vi "terminate.vi"(8 "error in (no error)":errorcluster, 11 "ExperimentControllerDL090803Triggered in":refnum<class "ExperimentControllerDL090803Triggered.lvclass">) -> (0 "error out":errorcluster, 3 "ExperimentControllerDL090803Triggered out":refnum<class "ExperimentControllerDL090803Triggered.lvclass">)   [LabVIEW 2010]
doc: "The dynamic dispatch version of this VI terminates the plug-in object by releasing all of its resources."
uses:
  ExperimentControllerDL090803Triggered.lvclass
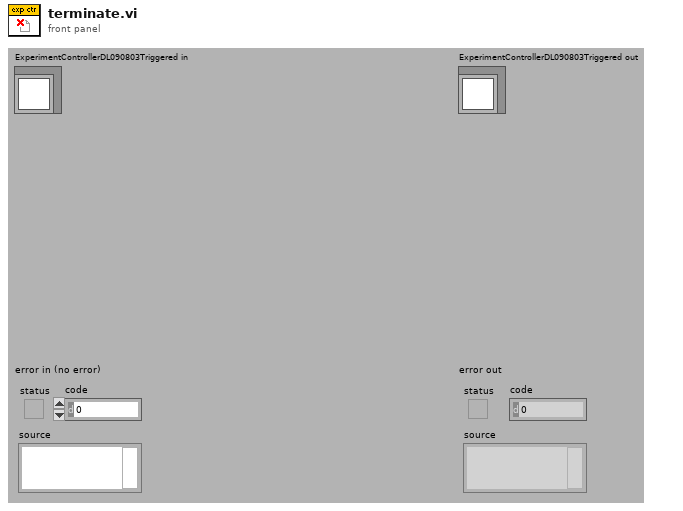
[diagram p1: front panel]
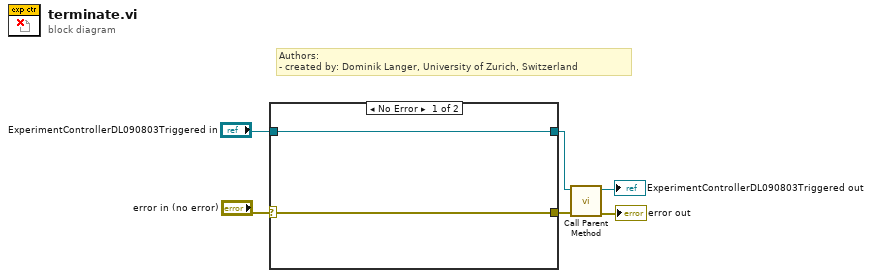
[diagram p0: block diagram]
diagram:
  # "Authors: \n- created by: Dominik Langer, University of Zurich, Switzerland"
  n1 = case shown="No Error" "error in (no error)" {
    selector: "error in (no error)" -> [w8 w10]
    tunnel: [w8 w10] -> w3
    tunnel: "ExperimentControllerDL090803Triggered in" -> [w7 w9]
    tunnel: [w7 w9] -> w2
    frame No Error {
    }
    frame Error {
    }
  }
  n2 = call-parent "Call Parent Method"("error in (no error)"=w3, "GenericPlugin in"=w2) -> ("error out"=→"error out":errorcluster, "GenericPlugin out"=→"ExperimentControllerDL090803Triggered out":refnum<class "ExperimentControllerDL090803Triggered.lvclass">)  [unwired: 8 out]
